vi "actuate_soultionChangeExp_v0.03.vi"(0 "Phase Cluster":T2, 1 "valve Time Cluster":T1, 2 "Didn't Lift?":bool, 3 "data in":T3={"daq_ao 1"="Dev1/ao0", "daq_ai 1"="Dev1/ai0", "experiment day folder"=path "D:/DATA/8-27-15 save func testing/test.lvm", "Multiclamp init error"=0, "Multiclamp Handle Out"=0, "sampling rate (Hz)"=10000, "trial name"=""}, 5 "PhaseLetter":string, 7 "controls array in":refnum<vi>[](array[refnum]), 9 "time to wait for solution change (min)":dbl=2.5 min=0.0 step=0.01, 11 "error in":errorcluster, 12 "common cluster":T6, 13 "individual controls in":T5) -> (4 "output cluster":T4={"daq_ao"="", "Duration (s)"=0.0, "Sample Freq (Hz)"=0.0, "Phase"=0.0, "Duty Cycle"=0.0, "Number of Replicates"=1} {"Number of Replicates" min=1 max=10}, 6 "protocol waveform":waveform(dbl)(graph), 8 "jumptestMonitor":waveform(dbl)[](graph) caption="protocol response", 10 "control array out":refnum<vi>[](array[refnum]), 14 "experiment VI ref":refnum<vi>, 15 "error out":errorcluster)   [LabVIEW 2019]
uses:
  pipette cleaning/pressure box/cleaning_soft/controls/actuator_type.ctl
  pipette cleaning/pressure box/cleaning_soft/controls/actuator_cluster.ctl
  machine_vision/coordinate model vis/transform_properties_actuators.ctl
  machine_vision/controls/transform_cluster_actuator.ctl
  controls/NH_method.ctl
  pipette cleaning/pressure box/cleaning_soft/controls/pressure_box_type.ctl
  pipette cleaning/pressure box/cleaning_soft/controls/pressure_box_control.ctl
  multipatch/controls/multipatch_common_controls_v4.ctl
  controls/memtest_def.ctl
  multipatch/controls/multipatch_individual_controls_v5.ctl
  Controls/Data.ctl
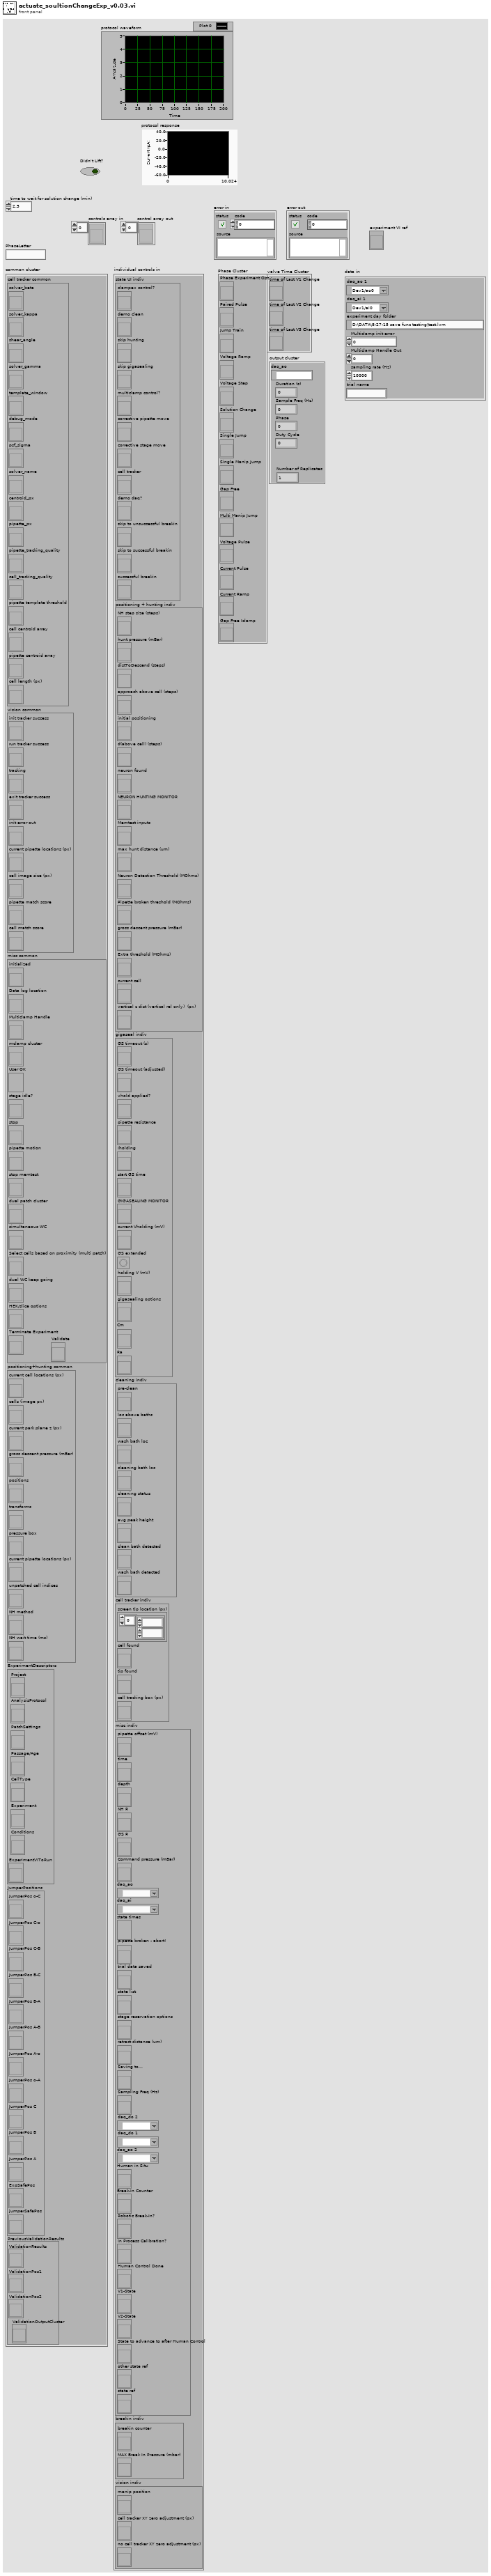
[diagram p1: front panel]
types:
  T1 = cluster{"time of Last V1 Change":refnum<vi>, "time of Last V2 Change":refnum<vi>, "time of Last V3 Change":refnum<vi>}
  T2 = cluster{"Phase Experiment Option":refnum<vi>, "Paired Pulse":refnum<vi>, "Jump Train":refnum<vi>, "Voltage Ramp":refnum<vi>, "Voltage Step":refnum<vi>, "Solution Change":refnum<vi>, "Single Jump":refnum<vi>, "Single Manip Jump":refnum<vi>, "Gap Free":refnum<vi>, "Multi Manip Jump":refnum<vi>, "Voltage Pulse":refnum<vi>, "Current Pulse":refnum<vi>, "Current Ramp":refnum<vi>, "Gap Free Iclamp":refnum<vi>}
  T3 = typedef "Data.ctl" = cluster{"daq_ao 1":tag, "daq_ai 1":tag, "experiment day folder":path, "Multiclamp init error":i32, "Multiclamp Handle Out":u32, "sampling rate (Hz)":i32, "trial name":string}
  T4 = cluster{"daq_ao":tag, "Duration (s)":dbl, "Sample Freq (Hz)":dbl, "Phase":dbl, "Duty Cycle":dbl, "Number of Replicates":i16}
  T5 = typedef "multipatch_individual_controls_v5.ctl" = cluster{"state UI indiv":cluster{"clampex control?":refnum<vi>, "demo clean":refnum<vi>, "skip hunting":refnum<vi>, "skip gigasealing":refnum<vi>, "multiclamp control?":refnum<vi>, "corrective pipette move":refnum<vi>, "corrective stage move":refnum<vi>, "cell tracker":refnum<vi>, "demo daq?":refnum<vi>, "skip to unsuccessful breakin":refnum<vi>, "skip to successful breakin":refnum<vi>, "successful breakin":refnum<vi>}, "positioning + hunting indiv":cluster{"NH step size (steps)":refnum<vi>, "hunt pressure (mBar)":refnum<vi>, "distToDescend (steps)":refnum<vi>, "approach above cell (steps)":refnum<vi>, "initial positioning":refnum<vi>, "d(above cell) (steps)":refnum<vi>, "neuron found":refnum<vi>, "NEURON HUNTING MONITOR":refnum<vi>, "Memtest inputs":refnum<vi>, "max hunt distance (um)":refnum<vi>, "Neuron Detection Threshold (MOhms)":refnum<vi>, "Pipette broken threshold (MOhms)":refnum<vi>, "gross descent pressure (mBar)":refnum<vi>, "Extra threshold (MOhms)":refnum<vi>, "current cell":refnum<vi>, "vertical z dist (vertical rel only)  (px)":refnum<vi>}, "gigaseal indiv":cluster{"GS timeout (s)":refnum<vi>, "GS timeout (adjusted)":refnum<vi>, "vhold applied?":refnum<vi>, "pipette resistance":refnum<vi>, "Iholding":refnum<vi>, "start GS time":refnum<vi>, "GIGASEALING MONITOR":refnum<vi>, "current Vholding (mV)":refnum<vi>, "GS extended":refnum<vi>, "holding V (mV)":refnum<vi>, "gigasealing options":refnum<vi>, "Cm":refnum<vi>, "Ra ":refnum<vi>}, "cleaning indiv":cluster{"pre-clean":refnum<vi>, "loc above baths":refnum<vi>, "wash bath loc":refnum<vi>, "cleaning bath loc":refnum<vi>, "cleaning status":refnum<vi>, "avg peak height":refnum<vi>, "clean bath detected":refnum<vi>, "wash bath detected":refnum<vi>}, "cell tracker indiv":cluster{"screen tip location (px)":refnum<vi>, "cell found":refnum<vi>, "tip found":refnum<vi>, "cell tracking box (px)":refnum<vi>}, "misc indiv":cluster{"pipette offset (mV)":refnum<vi>, "time":refnum<vi>, "depth":refnum<vi>, "NH R":refnum<vi>, "GS R":refnum<vi>, "Command pressure (mBar)":refnum<vi>, "daq_ao":tag, "daq_ai":tag, "state times":refnum<vi>, "pipette broken - abort!":refnum<vi>, "trial data saved":refnum<vi>, "state list":refnum<vi>, "stage reservation options":refnum<vi>, "retract distance (um)":refnum<vi>, "Saving to...":refnum<vi>, "Sampling Freq (Hz)":refnum<vi>, "daq_do 2":tag, "daq_do 1":tag, "daq_ao 2":tag, "Human in Situ":refnum<vi>, "Break-In Counter":refnum<vi>, "Robotic Break-In?":refnum<vi>, "In Process Calibration?":refnum<vi>, "Human Control Done":refnum<vi>, "V1-State":refnum<vi>, "V2-State":refnum<vi>, "State to advance to after Human Control":refnum<vi>, "other state ref":refnum<vi>, "state ref":refnum<vi>}, "breakin indiv":cluster{"breakin counter":refnum<vi>, "MAX Break In Pressure (mbar)":refnum<vi>}, "vision indiv":cluster{"manip position":refnum<vi>, "cell tracker XY zero adjustment (px)":refnum<vi>, "no cell tracker XY zero adjustment (px)":refnum<vi>}}
  T6 = typedef "multipatch_common_controls_v4.ctl" = cluster{"cell tracker common":cluster{"solver_beta":refnum<vi>, "solver_kappa":refnum<vi>, "shear_angle":refnum<vi>, "solver_gamma":refnum<vi>, "template_window":refnum<vi>, "debug_mode":refnum<vi>, "psf_sigma":refnum<vi>, "solver_name":refnum<vi>, "centroid_px":refnum<vi>, "pipette_px":refnum<vi>, "pipette_tracking_quality":refnum<vi>, "cell_tracking_quality":refnum<vi>, "pipette template threshold":refnum<vi>, "cell centroid array":refnum<vi>, "pipette centroid array":refnum<vi>, "cell length (px)":refnum<vi>}, "vision common":cluster{"init tracker success":refnum<vi>, "run tracker success":refnum<vi>, "tracking":refnum<vi>, "exit tracker success":refnum<vi>, "init error out":refnum<vi>, "current pipette locations (px)":refnum<vi>, "cell image size (px)":refnum<vi>, "pipette match score":refnum<vi>, "cell match score":refnum<vi>}, "misc common":cluster{"initialized":refnum<vi>, "Data log location":refnum<vi>, "Multiclamp Handle":refnum<vi>, "mclamp cluster":refnum<vi>, "User OK":refnum<vi>, "stage idle?":refnum<vi>, "stop":refnum<vi>, "pipette motion":refnum<vi>, "stop memtest":refnum<vi>, "dual patch cluster":refnum<vi>, "simultaneous WC":refnum<vi>, "Select cells based on proximity (multi patch)":refnum<vi>, "dual WC keep going":refnum<vi>, "HEK/slice options":refnum<vi>, "Terminate Experiment":refnum<vi>, "Validate":refnum<vi>}, "positioning+hunting common":cluster{"current cell locations (px)":refnum<vi>, "cells (image px)":refnum<vi>, "current park plane z (px)":refnum<vi>, "gross descent pressure (mBar)":refnum<vi>, "positions":refnum<vi>, "transforms":refnum<vi>, "pressure box":refnum<vi>, "current pipette locations (px)":refnum<vi>, "unpatched cell indices":refnum<vi>, "NH method":refnum<vi>, "NH wait time (ms)":refnum<vi>}, "ExperimentDescriptors":cluster{"Project":refnum<vi>, "AnalysisProtocol":refnum<vi>, "PatchSettings":refnum<vi>, "Passage/Age":refnum<vi>, "CellType":refnum<vi>, "Experiment":refnum<vi>, "Conditions":refnum<vi>, "ExperimentVIToRun":refnum<vi>}, "JumperPositions":cluster{"JumperPos o-C":refnum<vi>, "JumperPos C-o":refnum<vi>, "JumperPos C-B":refnum<vi>, "JumperPos B-C":refnum<vi>, "JumperPos B-A":refnum<vi>, "JumperPos A-B":refnum<vi>, "JumperPos A-o":refnum<vi>, "JumperPos o-A":refnum<vi>, "JumperPos C":refnum<vi>, "JumperPos B":refnum<vi>, "JumperPos A":refnum<vi>, "ExpSafePos":refnum<vi>, "jumperSafePos":refnum<vi>}, "PreviousValidationResults":cluster{"ValidationResults":refnum<vi>, "ValidationPos1":refnum<vi>, "ValidationPos2":refnum<vi>, "ValidationOutputCluster":refnum<vi>}}
  T7 = cluster{"Which Position to use for Experiment":enum16{"Jumper Safe Position", "Experiment Safe Position", "Jumper Position A", "Jumper Position B", "Jumper Position C", "Jumper Position o-A", "Jumper Position A-o", "Jumper Position A-B", "Jumper Position B-A", "Jumper Position B-C", "Jumper Position C-B", "Jumper Position C-o", "Jumper Position o-C", "Don't Move"}, "Duration (s)":dbl, "Delay (s)":dbl, "Pulse Width (s)":dbl, "Which Valve to Change?":i16, "Valve Jump Position":i16, "Replicates":dbl, "Vholding (mV)":dbl, "valve 1 used now?":bool, "valve 2 used now?":bool, "valve 3 used now? ":bool, "Valve 1 Position":i16, "Valve 2 Position":i16, "Valve 3 Position":i16, "protocol Preview":waveform(dbl)[]}
  T8 = enum16{"Jumper Safe Position", "Experiment Safe Position", "Jumper Position A", "Jumper Position B", "Jumper Position C", "Jumper Position o-A", "Jumper Position A-o", "Jumper Position A-B", "Jumper Position B-A", "Jumper Position B-C", "Jumper Position C-B", "Jumper Position C-o", "Jumper Position o-C", "Don't Move"}
  T9 = enum16{"manipulator 1", "manipulator 2", "manipulator 3", "manipulator 4"}
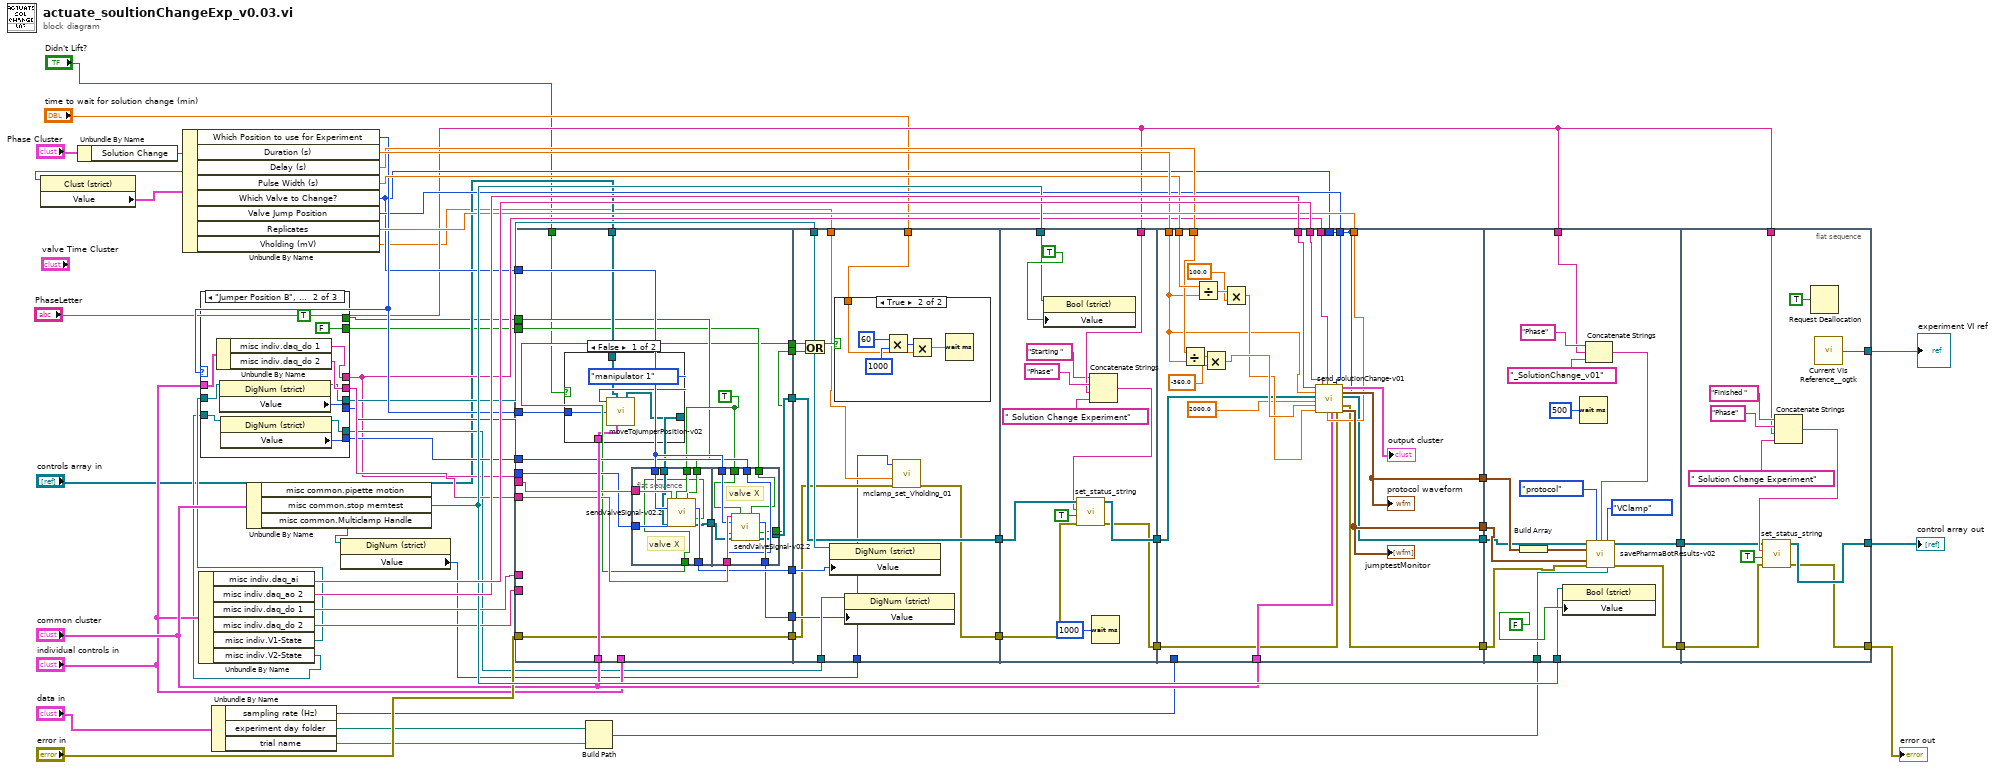
[diagram p0: block diagram]
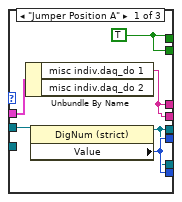
[diagram p2: hidden frame]
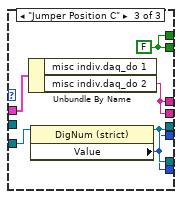
[diagram p3: hidden frame]
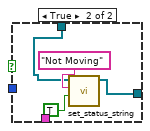
[diagram p4: hidden frame]
diagram:
  n1 = Unbundle By Name("Phase Cluster") -> ("Solution Change"=w41:refnum<vi>)
  n2 = property class="Clust (strict)"(reference=w41) -> ("Value"=w40:T7)  [unwired: 1 in, 2 out]
  n3 = Unbundle By Name(w40) -> ("Which Position to use for Experiment"=w33:T8, "Duration (s)"=w36:dbl, "Delay (s)"=w34:dbl, "Pulse Width (s)"=w35:dbl, "Which Valve to Change?"=w20:i16, "Valve Jump Position"=w21:i16, "Replicates"=w37:dbl, "Vholding (mV)"=w6:dbl)
  n4 = Unbundle By Name("individual controls in") -> ("misc indiv.daq_ai"=w59:tag, "misc indiv.daq_ao 2"=w58:tag, "misc indiv.daq_do 1"=w56:tag, "misc indiv.daq_do 2"=w55:tag, "misc indiv.V1-State"=w30:refnum<vi>, "misc indiv.V2-State"=w29:refnum<vi>)
  n5 = case shown="\"Jumper Position B\", Default" w33 {
    tunnel: "individual controls in" -> [w65 w76 w82]
    tunnel: [w64 w75 w81] -> w22
    tunnel: [w64 w74 w81] -> w31
    tunnel: w30 -> [w63 w73 _]
    tunnel: w29 -> [_ w70 w80]
    tunnel: [w62 w72 w78] -> w28
    tunnel: [w62 w68 w78] -> w27
    tunnel: [w61 w71 w79] -> w26
    tunnel: [w61 w69 w79] -> w24
    tunnel: [w60 TRUE w77] -> w10
    tunnel: [w60 FALSE w77] -> w9
    frame "Jumper Position A" {
      w60 = TRUE
      n6 = Unbundle By Name(w65) -> ("misc indiv.daq_do 1"=w64:tag)  [unwired: 1 out]
      n7 = property class="DigNum (strict)"(reference=w63) -> (reference out=w61:refnum<vi>, "Value"=w62:u16)  [unwired: 1 in, 1 out]
    }
    frame "Jumper Position B", Default {
      n8 = Unbundle By Name(w76) -> ("misc indiv.daq_do 1"=w75:tag, "misc indiv.daq_do 2"=w74:tag)
      n9 = property class="DigNum (strict)"(reference=w73) -> (reference out=w71:refnum<vi>, "Value"=w72:u16)  [unwired: 1 in, 1 out]
      n10 = property class="DigNum (strict)"(reference=w70) -> (reference out=w69:refnum<vi>, "Value"=w68:u16)  [unwired: 1 in, 1 out]
    }
    frame "Jumper Position C" {
      w77 = FALSE
      n11 = Unbundle By Name(w82) -> ("misc indiv.daq_do 2"=w81:tag)  [unwired: 1 out]
      n12 = property class="DigNum (strict)"(reference=w80) -> (reference out=w79:refnum<vi>, "Value"=w78:u16)  [unwired: 1 in, 1 out]
    }
  }
  n13 = Unbundle By Name("data in") -> ("sampling rate (Hz)"=w38:i32, "experiment day folder"=w46:path, "trial name"=w45:string)
  n14 = Unbundle By Name("common cluster") -> ("misc common.stop memtest"=w57:refnum<vi>, "misc common.Multiclamp Handle"=w5:refnum<vi>)  [unwired: 1 out]
  n15 = property class="DigNum (strict)"(reference=w5) -> ("Value"=w4:u32)  [unwired: 1 in, 2 out]
  n16 = flat-sequence {
    tunnel: "common cluster" -> [w102]
    tunnel: "individual controls in" -> [_]
    tunnel: w56 -> [_]
    tunnel: w55 -> [_]
    tunnel: "error in" -> [w101]
    tunnel: [w101] -> w50
    tunnel: w33 -> [w100]
    tunnel: w22 -> [w99]
    tunnel: w31 -> [w98]
    tunnel: w20 -> [w97]
    tunnel: w28 -> [w96]
    tunnel: w27 -> [w95]
    tunnel: [w94] -> w25
    tunnel: [w93] -> w23
    tunnel: "controls array in" -> [w92]
    tunnel: [w89] -> w15
    tunnel: w10 -> [w87]
    tunnel: w9 -> [w86]
    tunnel: [w85] -> w8
    tunnel: [w84] -> w7
    tunnel: "Didn't Lift?" -> [w83]
    tunnel: [w131] -> w51
    tunnel: w50 -> [w134]
    tunnel: w26 -> [w142]
    tunnel: w25 -> [w141]
    tunnel: w24 -> [w140]
    tunnel: w23 -> [w139]
    tunnel: [w138] -> w16
    tunnel: w15 -> [w138]
    tunnel: w8 -> [w136]
    tunnel: w7 -> [w135]
    tunnel: w6 -> [w133]
    tunnel: w4 -> [w132]
    tunnel: "time to wait for solution change (min)" -> [w130]
    tunnel: w57 -> [w158]
    tunnel: [w154] -> w52
    tunnel: w51 -> [w155]
    tunnel: [w156] -> w17
    tunnel: w16 -> [w157]
    tunnel: "PhaseLetter" -> [w149]
    tunnel: w59 -> [w184]
    tunnel: w58 -> [w183]
    tunnel: [w164] -> w53
    tunnel: w52 -> [w165]
    tunnel: [w181] -> w49
    tunnel: [w180] -> w48
    tunnel: "common cluster" -> [w166]
    tunnel: [w167] -> _
    tunnel: w36 -> [w171]
    tunnel: w35 -> [w175]
    tunnel: w34 -> [w174]
    tunnel: w38 -> [_]
    tunnel: w37 -> [w170]
    tunnel: w22 -> [w169]
    tunnel: w21 -> [w168]
    tunnel: w20 -> [w167]
    tunnel: [w162] -> w18
    tunnel: w17 -> [w163]
    tunnel: w57 -> [w200]
    tunnel: w53 -> [w189]
    tunnel: w49 -> [w199]
    tunnel: w48 -> [w197]
    tunnel: w44 -> [w194]
    tunnel: "PhaseLetter" -> [w190]
    tunnel: w18 -> [w188]
    tunnel: [w186] -> w13
    tunnel: [w187] -> w12
    tunnel: [w207] -> w14
    tunnel: [w205] -> w42
    tunnel: w13 -> [w206]
    tunnel: w12 -> [w208]
    tunnel: "PhaseLetter" -> [w204]
    tunnel: [w203] -> w1
    frame #0 {
      w88 = TRUE
      n17 = case shown="False" w83 {
        tunnel: w102 -> [w107 _]
        tunnel: w100 -> [w105 _]
        tunnel: w92 -> [w104 w109]
        tunnel: [w103 w110] -> w91
        frame False {
          n18 = call "moveToJumperPosition-v02.vi"("which manipulator"=T9."manipulator 1", "controls array in"=w104, "Which Jumper Position to move to?"=w105, "common cluster"=w107) -> ("control array out"=w103:refnum<vi>[])  [unwired: 10 in, 1 out]
        }
        frame True {
          n19 = call "set_status_string.vi"("new line?"=TRUE, "status string in"="Not Moving", "controls array"=w109) -> ("controls array out"=w110:refnum<vi>[])  [unwired: 7 in, 1 out]
        }
      }
      n20 = flat-sequence {
        tunnel: [w120] -> w94
        tunnel: w99 -> [w119]
        tunnel: w97 -> [w118]
        tunnel: w96 -> [w117]
        tunnel: w91 -> [w116]
        tunnel: [w115] -> w90
        tunnel: w88 -> [w114]
        tunnel: w87 -> [w113]
        tunnel: [w112] -> w84
        tunnel: w98 -> [w129]
        tunnel: w97 -> [w128]
        tunnel: [w127] -> w93
        tunnel: w95 -> [w126]
        tunnel: w90 -> [w125]
        tunnel: [w124] -> w89
        tunnel: w88 -> [w123]
        tunnel: w86 -> [w122]
        tunnel: [w121] -> w85
        frame #0 {
          # "valve X"
          n21 = call "sendValveSignal-v02.2.vi"("daq_do"=w119, "Valve1?"=w113, "ChangeToValve"=w118, "CurrentValve"=w117, "controls array in"=w116, "Set Status"=w114) -> ("ValveSetTo"=w120:u16, "valve changed?"=w112:bool, "control array out"=w115:refnum<vi>[])  [unwired: 6 in, 1 out]
        }
        frame #1 {
          # "valve X"
          n22 = call "sendValveSignal-v02.2.vi"("daq_do"=w129, "Valve1?"=w122, "ChangeToValve"=w128, "CurrentValve"=w126, "controls array in"=w125, "Set Status"=w123) -> ("ValveSetTo"=w127:u16, "valve changed?"=w121:bool, "control array out"=w124:refnum<vi>[])  [unwired: 6 in, 1 out]
        }
      }
    }
    frame #1 {
      n23 = Or(x=w135, y=w136) -> (x .or. y?=w137:bool)
      n24 = property class="DigNum (strict)"(reference=w142, "Value"=w141) -> ()  [unwired: 1 in, 2 out]
      n25 = case shown="True" w137 {
        tunnel: w130 -> [_ w143]
        frame False {
        }
        frame True {
          n26 = Multiply(x=u32 60 ("milliseconds to wait"), y=u32 1000) -> (x*y=w145:u32)
          n27 = Multiply(x=w145, y=w143) -> (x*y=w144:dbl)
          n28 = Wait (ms)(milliseconds to wait=w144) -> ()  [unwired: 1 out]
        }
      }
      n29 = property class="DigNum (strict)"(reference=w140, "Value"=w139) -> ()  [unwired: 1 in, 2 out]
      n30 = call "mclamp_set_Vholding_01.vi"("error in (no error)"=w134, "set holding (mV)"=w133, "Multiclamp Handle Out"=w132) -> ("error out"=w131:errorcluster)  [unwired: 7 in, 1 out]
    }
    frame #2 {
      n31 = property class="Bool (strict)"(reference=w158, "Value"=TRUE ("stop memtest")) -> ()  [unwired: 1 in, 2 out]
      n32 = Concatenate Strings("Starting " ("string"), "Phase" ("string"), w149, " Solution Change Experiment" ("string")) -> (w150:string)
      n33 = call "set_status_string.vi"("error in"=w155, "new line?"=TRUE, "status string in"=w150, "controls array"=w157) -> ("error out"=w154:errorcluster, "controls array out"=w156:refnum<vi>[])  [unwired: 6 in]
      n34 = Wait (ms)(milliseconds to wait=u32 1000) -> ()  [unwired: 1 out]
    }
    frame #3 {
      n35 = Divide(x=w174, y=w171) -> (x/y=w176:dbl)
      n36 = Divide(x=w175, y=w171) -> (x/y=w179:dbl)
      n37 = Multiply(x=w176, y=-360.0) -> (x*y=w173:dbl)
      n38 = Multiply(x=w179, y=100.0) -> (x*y=w172:dbl)
      n39 = call "send_solutionChange-v01.vi"("daq_ao 2"=w183, "Duration (s)"=w171, "controls array in"=w163, "Sample Freq (Hz)"=2000.0, "Phase"=w173, "Duty Cycle"=w172, "daq_ai"=w184, "daq_do"=w169, "Number of Replicates"=w170, "Start Position"=w167, "common cluster"=w166, "Jump Position"=w168, "error in"=w165) -> ("output cluster"=→"output cluster":T4, "output waveform"=w181:waveform(dbl), "control array out"=w162:refnum<vi>[], "error out"=w164:errorcluster, "jumptestMonitor"=w180:waveform(dbl)[])  [unwired: 2 in]
      "jumptestMonitor" <- w180
      "protocol waveform" <- w181
    }
    frame #4 {
      n40 = Build Array(w199) -> (w198:waveform(dbl)[])
      n41 = property class="Bool (strict)"(reference=w200, "Value"=FALSE ("stop memtest")) -> ()  [unwired: 1 in, 2 out]
      n42 = Wait (ms)(milliseconds to wait=u32 500) -> ()  [unwired: 1 out]
      n43 = Concatenate Strings("Phase" ("string"), w190, "_SolutionChange_v01" ("string")) -> (w191:string)
      n44 = call "savePharmaBotResults-v02.vi"("controls array"=w188, "protocol or memtest"=enum16{"protocol", "memtest", "validation"}."protocol", "ExpPhase"=w191, "which clamp"=enum16{"VClamp", "IClamp"}."VClamp", "protocol waveform"=w198, "protocol response"=w197, "error in"=w189, "Save to (folder dir)"=w194) -> ("controls array out"=w187:refnum<vi>[], "error out"=w186:errorcluster)  [unwired: 6 in]
    }
    frame #5 {
      n45 = Concatenate Strings("Finished " ("string"), "Phase" ("string"), w204, " Solution Change Experiment" ("string")) -> (w210:string)
      n46 = call "set_status_string.vi"("error in"=w206, "new line?"=TRUE, "status string in"=w210, "controls array"=w208) -> ("error out"=w205:errorcluster, "controls array out"=w207:refnum<vi>[])  [unwired: 6 in]
      n47 = Request Deallocation(TRUE ("flag")) -> ()
      n48 = call "Current VIs Reference__ogtk.vi"() -> ("Current VI's reference"=w203:refnum<vi>)  [unwired: 5 in]
    }
  }
  n49 = Build Path(base path=w46, name or relative path=w45) -> (appended path=w44:path)
  "error out" <- w42
  "control array out" <- w14
  "experiment VI ref" <- w1
